vi "draw an ellipse V2.vi"(4 "ellipse factor":dbl=10.0, 6 "number of points":i32=20, 8 "2D curvature tensor IN":T1={"curvature Matrix"=[[3.0, 1.0], [1.0, 4.0]], "Eigenvalues"=[4.618033988749895+0.0i, 2.381966011250105+0.0i], "Eigenvectors"=[[-0.8506508083520399+0.0i, -0.5257311121191335+0.0i], [0.5257311121191335+0.0i, -0.8506508083520399+0.0i]], "theta (rad)"=0.5535743588970453+0.0i, "theta (deg)"=31.717474411461012+0.0i, "sigmas"=[4.618033988749895+0.0i, 2.381966011250105+0.0i]}, 10 "2D curvature Matrix IN":T2, 11 "center IN":cluster{"center x":dbl, "center Y":dbl}) -> (0 "2D curvature tensor OUT":T1={"curvature Matrix"=[[3.0, 1.0], [1.0, 4.0]], "Eigenvalues"=[4.618033988749895+0.0i, 2.381966011250105+0.0i], "Eigenvectors"=[[-0.8506508083520399+0.0i, -0.5257311121191335+0.0i], [0.5257311121191335+0.0i, -0.8506508083520399+0.0i]], "theta (rad)"=0.5535743588970453+0.0i, "theta (deg)"=31.717474411461012+0.0i, "sigmas"=[4.618033988749895+0.0i, 2.381966011250105+0.0i]}, 2 "2D curvature Matrix OUT":T2=[[3.0, 1.0], [1.0, 4.0]], 3 "ellipse OUT":cluster{"Array":dbl[], "Array":dbl[]})   [LabVIEW 2020]
uses:
  <vilib>/Analysis/Matrix/Datatypes/RealMatrix.ctl
  2D curvature tensor.ctl
  <vilib>/Analysis/Matrix/Datatypes/ComplexMatrix.ctl
  array -- bilinear regression 2D.ctl
  array of vectors -- algebra.ctl
  2D curvature tensor actions.ctl
  generate linear region.vi
  <vilib>/Analysis/7linalg.llb/Eigenvalues and Vectors.vi
  <vilib>/Analysis/7linalg.llb/Real Eigenvalues and Vectors.vi
  <vilib>/Analysis/Matrix/NI_Matrix.lvlib
panel:
  out "sigmatau":cluster{"Numeric":dbl, "Numeric":dbl}
  out "Plot: curvature":cluster{dbl[], dbl[]}(graph)
  out "z out":dbl[](array[numeric])
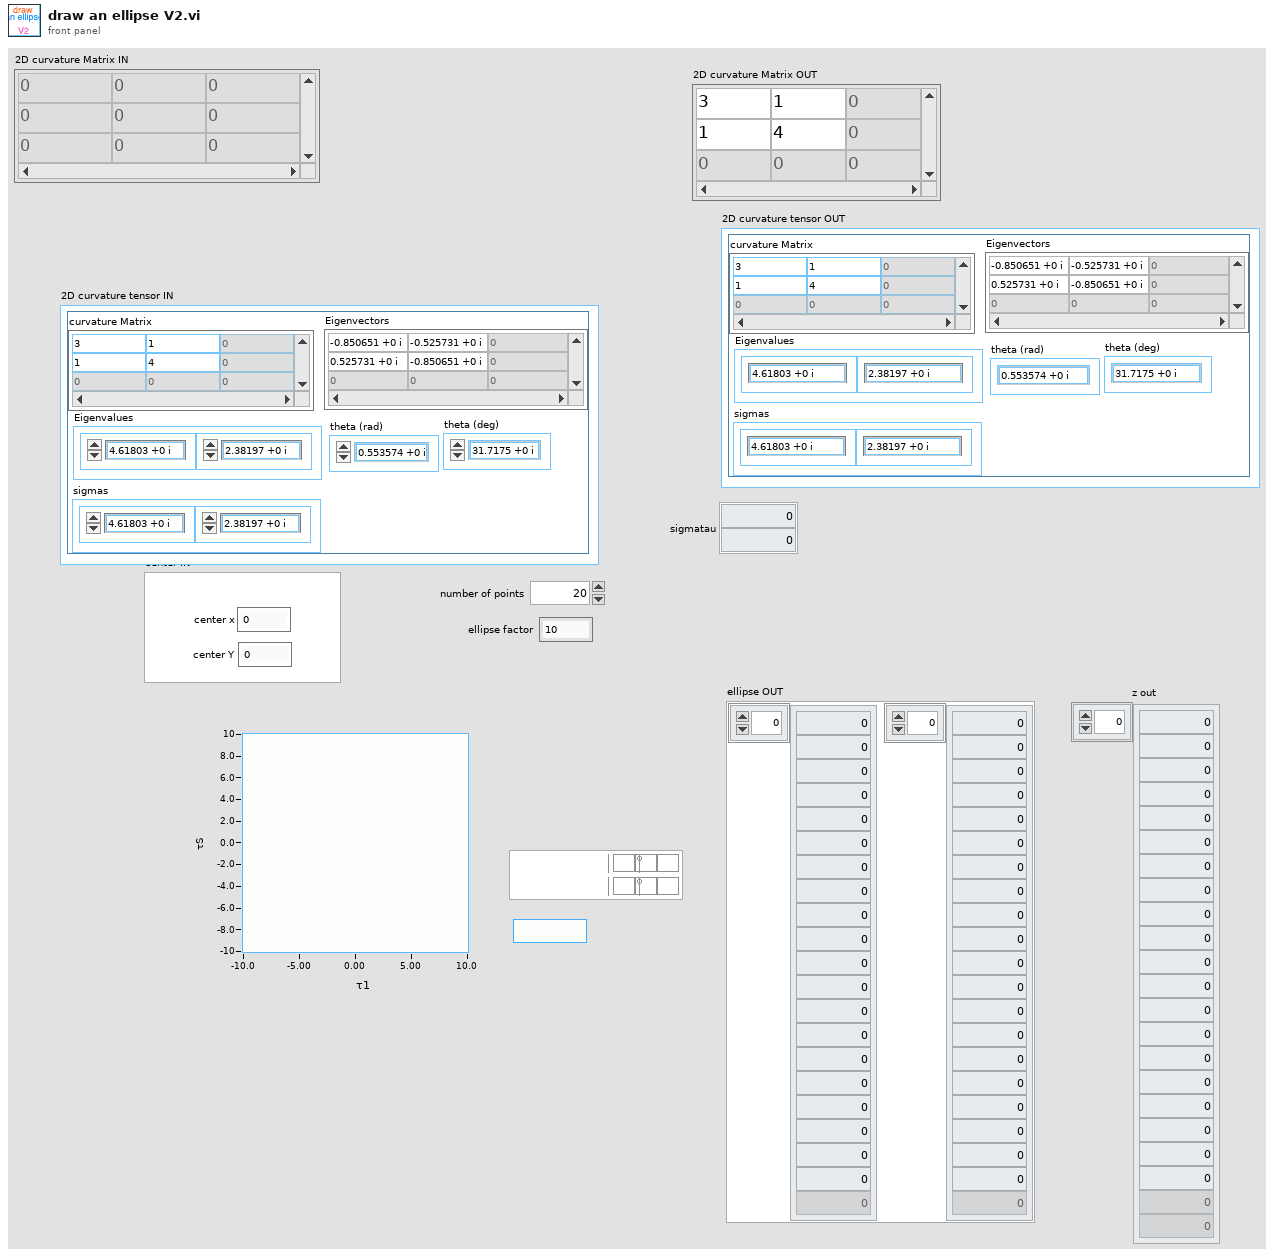
[diagram p1: front panel]
types:
  T1 = typedef "2D curvature tensor.ctl" = cluster{"curvature Matrix":T2, "Eigenvalues":cdb[], "Eigenvectors":T3, "theta (rad)":cdb, "theta (deg)":cdb, "sigmas":cdb[]}
  T2 = typedef "NI_Matrix.lvlib/RealMatrix.ctl" = dbl[][]
  T3 = typedef "NI_Matrix.lvlib/ComplexMatrix.ctl" = cdb[][]
  T4 = typedef "2D curvature tensor actions.ctl" = enum16{"eigensystem", "sigma", "set matrix"}
  T5 = typedef "array of vectors -- algebra.ctl" = enum16{"shift", "rotate", "scale", "multiply", "expectation"}
  T6 = typedef "array -- bilinear regression 2D.ctl" = enum16{"1", "x", "y", "xx", "xy", "yy", "xxy", "xyy", "yyy", "xxx", "xxyy", "xyyy", "xxxy", "yyyy", "xxxx", "xxz", "xyz", "yyz", "xz", "yz", "z"}
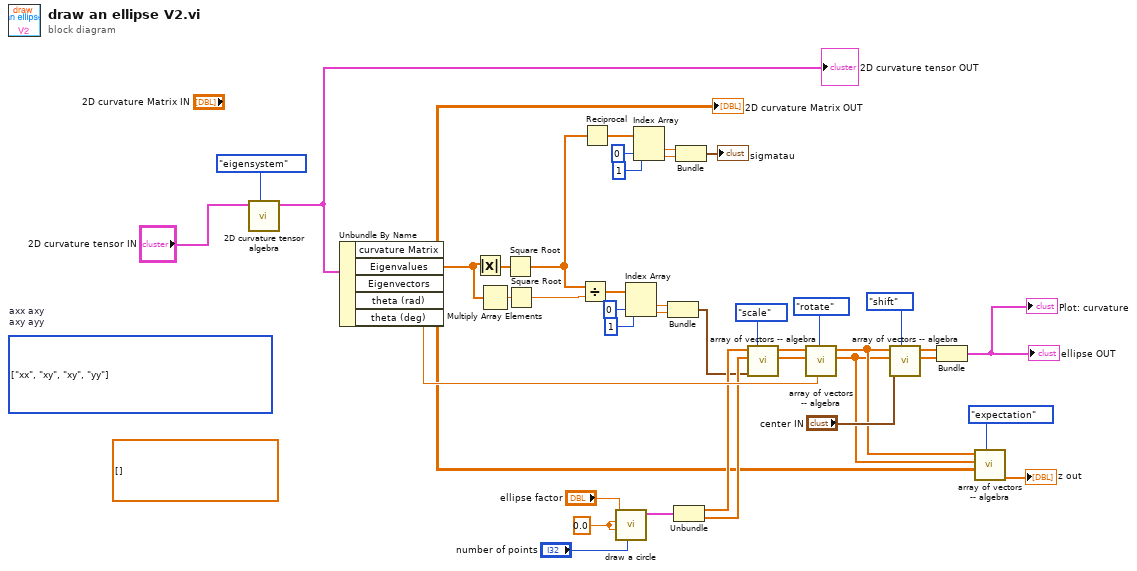
[diagram p0: block diagram]
diagram:
  (unwired) T2 [] ("curvature Matrix IN")
  (unwired) T6[][] [[enum."xx", enum."xy"], [enum."xy", enum."yy"]] items=["1", "x", "y", "xx", "xy", "yy", "xxy", "xyy", "yyy", "xxx", "xxyy", "xyyy", "xxxy", "yyyy", "xxxx", "xxz", "xyz", "yyz", "xz", "yz", "z"]  # axx axy axy ayy
  w39 = 0.0 ("center x")
  n1 = call "2D curvature tensor algebra.vi"("2D tensor"=2D_curvature_tensor_actions."eigensystem", "curvature tensor IN"="2D curvature tensor IN") -> ("curvature tensor OUT"=w2:T1)  [unwired: 7 in, 2 out]
  "2D curvature tensor OUT" <- w2
  n2 = Unbundle By Name(w2) -> ("curvature Matrix"=w4:T2, "Eigenvalues"=w34:cdb[], "theta (rad)"=w30:cdb)  [unwired: 2 out]
  "2D curvature Matrix OUT" <- w4
  n3 = Absolute Value(x=w34) -> (abs(x)=w37:dbl[])
  n4 = Multiply Array Elements(1:w34) -> (0:w35:cdb)
  n5 = Square Root ("Square Root.vi")(x=w37) -> (sqrt(x)=w7:dbl[])
  n6 = Square Root(x=w35) -> (sqrt(x)=w33:cdb)
  n7 = Divide(x=w7, y=w33) -> (x/y=w26:cdb[])
  n8 = Reciprocal(x=w7) -> (1/x=w6:dbl[])
  n9 = call "draw a circle.vi"("number of points"="number of points", "center Y"=w39, "center x"=w39, "radius"="ellipse factor") -> ("output cluster"=w40:cluster{dbl[], dbl[]})  [unwired: 7 in]
  n10 = Index Array(array=w26, index #1=0 ("index"), index #2=1 ("index")) -> (element #1=w20:cdb, element #2=w21:cdb)
  n11 = Index Array(array=w6, index #1=0 ("index"), index #2=1 ("index")) -> (element #1=w8:dbl, element #2=w9:dbl)
  n12 = Bundle(w20, w21) -> (w19:cluster{cdb, cdb})  [unwired: 1 in]
  n13 = Unbundle(w40) -> (w28:dbl[], w27:dbl[])
  n14 = Bundle("Numeric"=w8, "Numeric"=w9) -> (→"sigmatau":cluster{"Numeric":dbl, "Numeric":dbl})  [unwired: 1 in]
  n15 = call "array of vectors -- algebra.vi"("Enum"=array_of_vectors_--_algebra."scale", "vec IN"=w19, "y IN"=w27, "x IN"=w28) -> ("y IOUT"=w22:dbl[], "x  OUT"=w23:dbl[])  [unwired: 5 in, 1 out]
  n16 = call "array of vectors -- algebra.vi"("theta"=w30, "Enum"=array_of_vectors_--_algebra."rotate", "y IN"=w22, "x IN"=w23) -> ("y IOUT"=w13:dbl[], "x  OUT"=w14:dbl[])  [unwired: 5 in, 1 out]
  n17 = call "array of vectors -- algebra.vi"("Enum"=array_of_vectors_--_algebra."shift", "vec IN"="center IN", "y IN"=w13, "x IN"=w14) -> ("y IOUT"=w16:dbl[], "x  OUT"=w17:dbl[])  [unwired: 5 in, 1 out]
  n18 = Bundle("x  OUT"=w17, "y IOUT"=w16) -> (→"ellipse OUT" →"Plot: curvature":cluster{"x  OUT":dbl[], "y IOUT":dbl[]})  [unwired: 1 in]
  n19 = call "array of vectors -- algebra.vi"("Enum"=array_of_vectors_--_algebra."expectation", "Matrix"=w4, "y IN"=w13, "x IN"=w14) -> ("z out"=→"z out":dbl[])  [unwired: 5 in, 2 out]
